vi "CMD_VERSION.vi"(8 "error in (no error)":errorcluster, 10 "Arguments":string[](array[string]), 11 "gScript Interpreter in":refnum<class "gScript Interpreter.lvclass">) -> (0 "error out":errorcluster, 3 "gScript Interpreter out":refnum<class "gScript Interpreter.lvclass">)   [LabVIEW 2023, in "gScript Interpreter.lvclass"]
uses:
  gScript Interpreter.lvclass
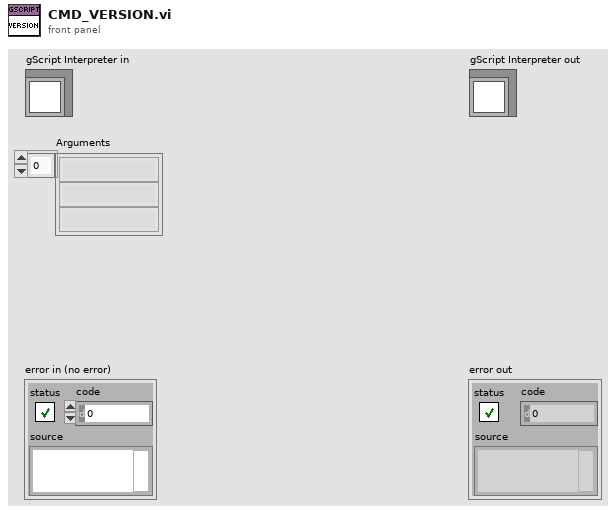
[diagram p1: front panel]
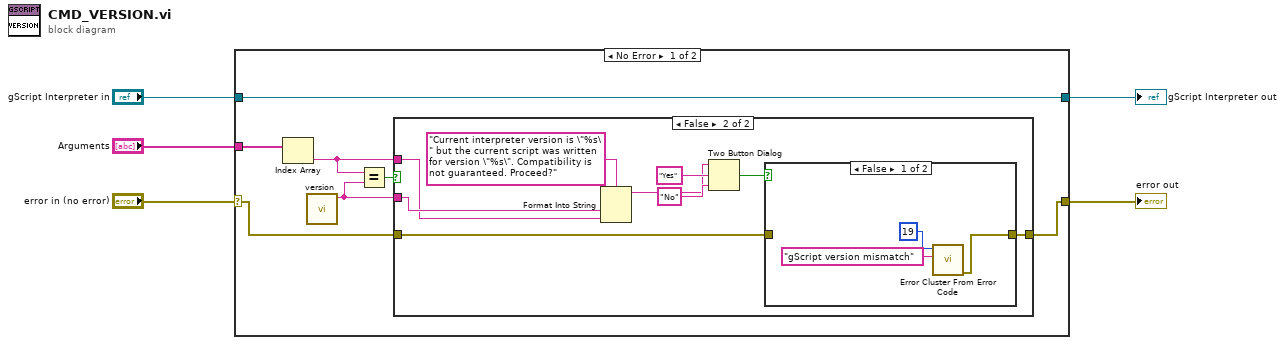
[diagram p0: block diagram]
diagram:
  n1 = case shown="No Error" "error in (no error)" {
    selector: "error in (no error)" -> [w9 w28]
    tunnel: [w8 w28] -> w4
    tunnel: [w11 w27] -> w2
    tunnel: "gScript Interpreter in" -> [w11 w27]
    tunnel: "Arguments" -> [w12 _]
    frame No Error {
      n2 = Index Array(array=w12) -> (element=w6:string)  [unwired: 1 in]
      n3 = call "version.vi"() -> ("Version"=w7:string)  [unwired: 3 in]
      n4 = Equal?(x=w6, y=w7) -> (x = y?=w10:bool)
      n5 = case shown="False" w10 {
        tunnel: w9 -> [w13 w15]
        tunnel: [w13 w14] -> w8
        tunnel: w7 -> [_ w18]
        tunnel: w6 -> [_ w17]
        frame True {
        }
        frame False {
          n6 = Format Into String(format string="Current interpreter version is \"%s\" but the current script was written for version \"%s\". Compatibility is not guaranteed. Proceed?", w18, w17) -> (resulting string=w19:string)  [unwired: 2 in, 1 out]
          n7 = Two Button Dialog(message=w19, 1:"No" ("t"), 2:"Yes" ("t")) -> (T button?=w16:bool)
          n8 = case shown="False" w16 {
            tunnel: w15 -> [_ w26]
            tunnel: [w23 w26] -> w14
            frame False {
              n9 = call <vilib>:"Error Cluster From Error Code.vi"("error message (\"\")"="gScript version mismatch" ("error message (\"\")"), "error code (0)"=19) -> ("error out"=w23:errorcluster)  [unwired: 7 in]
            }
            frame True {
            }
          }
        }
      }
    }
    frame Error {
    }
  }
  "error out" <- w4
  "gScript Interpreter out" <- w2
